vi "calculate_extinction_center_xi_zero.vi"(8 "Error In":errorcluster, 11 "Xtal Description":T1) -> (0 "Error Out":errorcluster, 3 "prediction":dbl)   [LabVIEW 2019]
uses:
  xtal_description_for_prediction_cluster_typedef.ctl
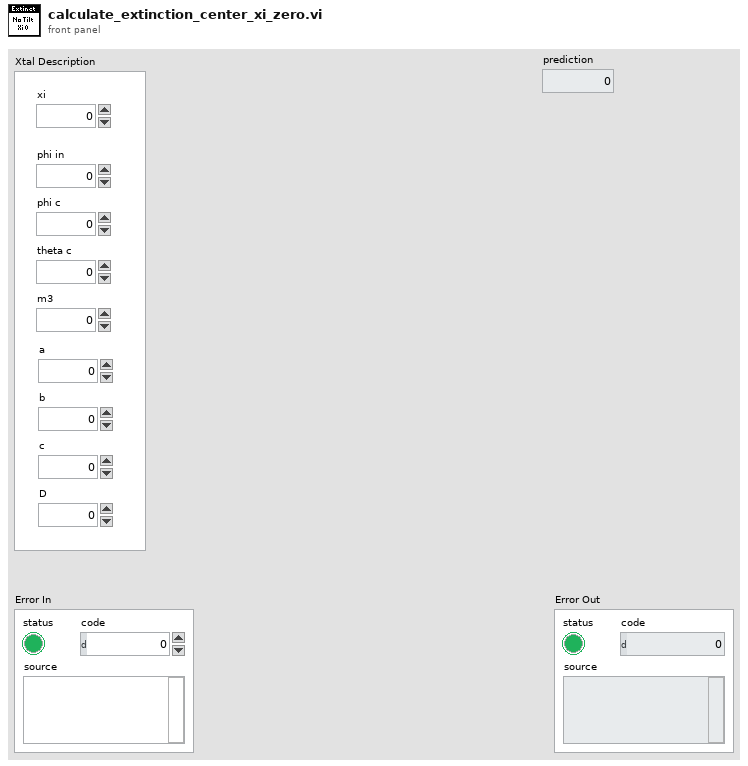
[diagram p1: front panel]
types:
  T1 = typedef "xtal_description_for_prediction_cluster_typedef.ctl" = cluster{"xi":dbl, "phi in":dbl, "phi c":dbl, "theta c":dbl, "m3":dbl, "a":dbl, "b":dbl, "c":dbl, "D":dbl}
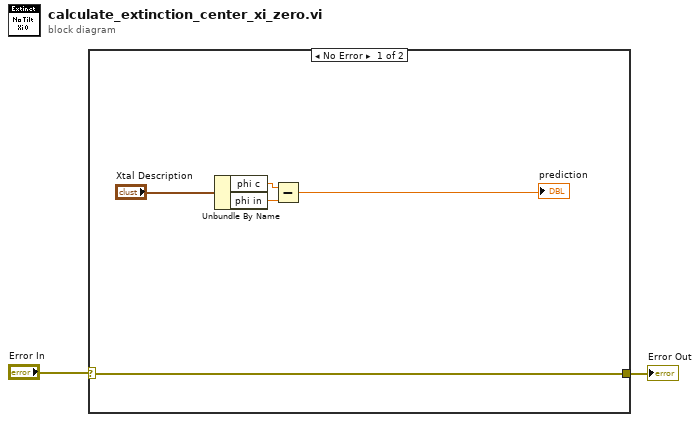
[diagram p0: block diagram]
diagram:
  n1 = case shown="No Error" "Error In" {
    selector: "Error In" -> [w7 w8]
    tunnel: [w7 w8] -> w1
    frame No Error {
      n2 = Unbundle By Name("Xtal Description") -> ("phi c"=w4:dbl, "phi in"=w5:dbl)
      n3 = Subtract(x=w4, y=w5) -> (x-y=→"prediction":dbl)
    }
    frame Error {
    }
  }
  "Error Out" <- w1
